vi "ROI_positions_embryo_SAVE.vi"(2 "XY positions":dbl[][](array[numeric]), 4 "error in":errorcluster) -> (0 "error out":errorcluster, 1 "XY positions OUT":dbl[][](array[numeric]))   [LabVIEW 2015]
uses:
  GLOBAL/Global_MAIN.vi
  GLOBAL/Global_ASI_stage.vi
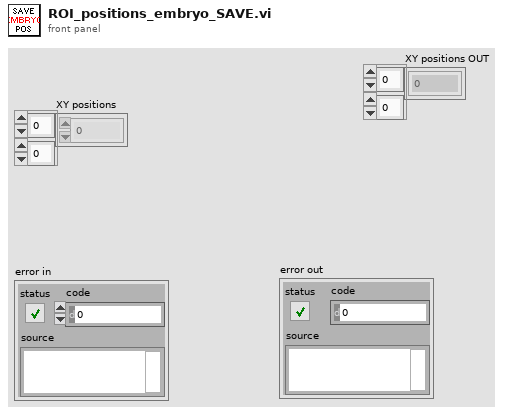
[diagram p1: front panel]
types:
  T1 = enum16{"open", "open or create", "create or replace", "create", "open (read-only)"}
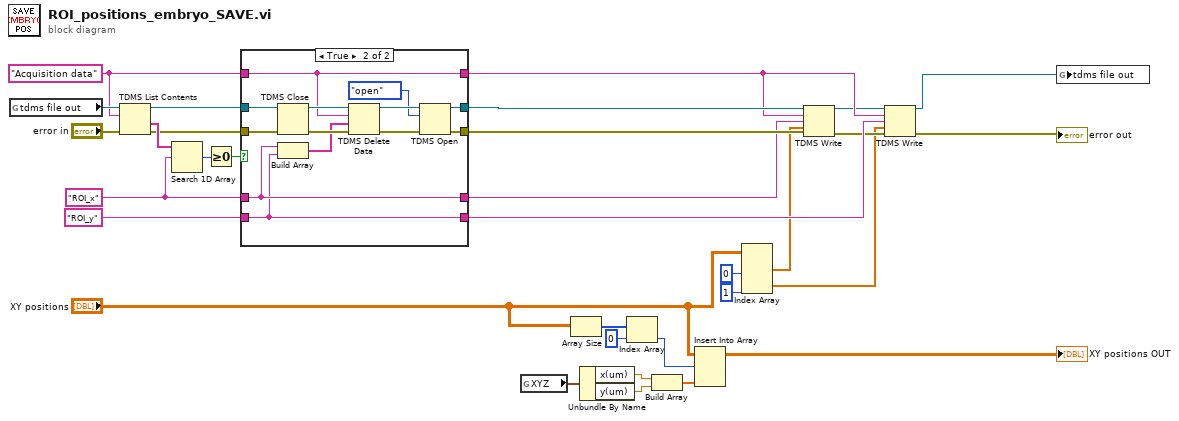
[diagram p0: block diagram]
diagram:
  w19 = "ROI_x"
  w20 = "Acquisition data" ("group name in (Untitled)")
  n1 = global read "Global_MAIN.vi" "tdms file out"() -> (w23:refnum<k34>)
  n2 = TDMS List Contents(4:"error in", 6:w20, 7:w23) -> (0:w18:errorcluster, 1:w24:string[], 3:w21:refnum<k34>)  [unwired: 1 out]
  n3 = Search 1D Array(1D array=w24, element=w19) -> (index of element=w25:i32)  [unwired: 1 in]
  n4 = Greater Or Equal To 0?(x=w25) -> (x >= 0?=w17:bool)
  n5 = case shown="True" w17 {
    tunnel: "ROI_y" -> [w34 w39]
    tunnel: [w37 w44] -> w28
    tunnel: [w36 w43] -> w27
    tunnel: w21 -> [w37 w42]
    tunnel: w20 -> [w33 w38]
    tunnel: w19 -> [w35 w40]
    tunnel: w18 -> [w36 w41]
    tunnel: [w35 w40] -> w16
    tunnel: [w34 w39] -> w15
    tunnel: [w33 w38] -> w14
    frame False {
    }
    frame True {
      n6 = TDMS Close(8:w41, 11:w42) -> (0:w49:errorcluster, 3:w50:path)
      n7 = Build Array(w40, w39) -> (w48:string[])
      n8 = TDMS Delete Data(8:w49, 9:w48, 10:w38, 11:w50) -> (0:w46:errorcluster, 3:w47:path)  [unwired: 3 in]
      n9 = TDMS Open(8:w46, 10:T1."open" ("operation (0:open)"), 11:w47) -> (0:w43:errorcluster, 3:w44:refnum<k34>)  [unwired: 4 in]
    }
  }
  n10 = global read "Global_ASI_stage.vi" "XYZ"() -> (w9:cluster{"x(um)":dbl, "y(um)":dbl, "z(um)":dbl})
  n11 = Array Size(array="XY positions") -> (size(s)=w10:i32[])
  n12 = Unbundle By Name(w9) -> ("x(um)"=w8:dbl, "y(um)"=w7:dbl)
  n13 = Index Array(array=w10, index=0) -> (element=w12:i32)
  n14 = Build Array(w8, w7) -> (w13:dbl[])
  n15 = Insert Into Array(array="XY positions", index (row)=w12, new element=w13) -> (→"XY positions OUT":dbl[][])  [unwired: 1 in]
  n16 = Index Array(array="XY positions", index (col) #1=0 ("disabled index (col)"), index (col) #2=1 ("index (col)")) -> (element #1=w5:dbl[], element #2=w2:dbl[])  [unwired: 2 in]
  n17 = TDMS Write(0:w28, 5:w14, 7:w16, 9:w5, 11:w27) -> (4:w1:refnum<k34>, 15:w4:errorcluster)  [unwired: 1 in, 2 out]
  n18 = TDMS Write(0:w1, 5:w14, 7:w15, 9:w2, 11:w4) -> (4:w26:refnum<k34>, 15:→"error out":errorcluster)  [unwired: 1 in, 2 out]
  n19 = global write "Global_MAIN.vi" "tdms file out"(w26) -> ()
